vi "rs3 free error.vi"(8 "error in (no error)":errorcluster, 11 "error in":u64) -> (0 "error out 2":errorcluster, 3 "error out":u64)   [LabVIEW 2023]
doc: "void rs_free_error (rs_error * error);"
uses:
  realsense2.dll
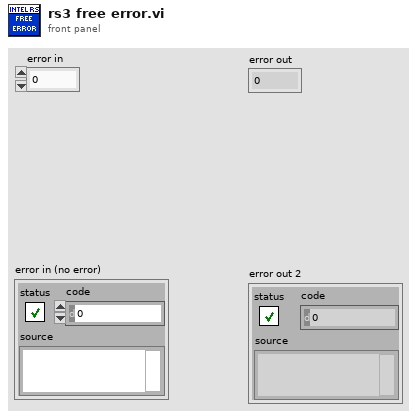
[diagram p1: front panel]
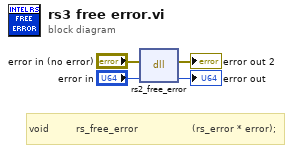
[diagram p0: block diagram]
diagram:
  # "void         rs_free_error                  (rs_error * error);"
  n1 = dll-call lib="C:/STEAMSyndicate/RealSenseWrappers/VI Wrappers (add ons) Public/RealSense/realsense2.dll" fn="rs2_free_error"(error in="error in (no error)", "error"="error in") -> (error out=→"error out 2":errorcluster, "error"=→"error out":u64)  [unwired: 3 in, 1 out]
